vi "Start Sync.vi"(8 "error in (no error)":errorcluster, 11 "gRPC service in":refnum<class "OOBgRPCService.lvclass">) -> (0 "error out":errorcluster, 3 "gRPC service out":refnum<class "OOBgRPCService.lvclass">)   [LabVIEW 2025, in "OOB gRPC Server.lvlib" / "OOBgRPCService.lvclass"]
uses:
  OOBgRPCService.lvclass
  OOBgRPCService.lvclass/OOBgRPCService.ctl
  OOB Data Transfer/OOB Data Transfer.lvlib
  RPC Messages/hwval_GenericResponse.ctl
  OOB gRPC Server.lvlib
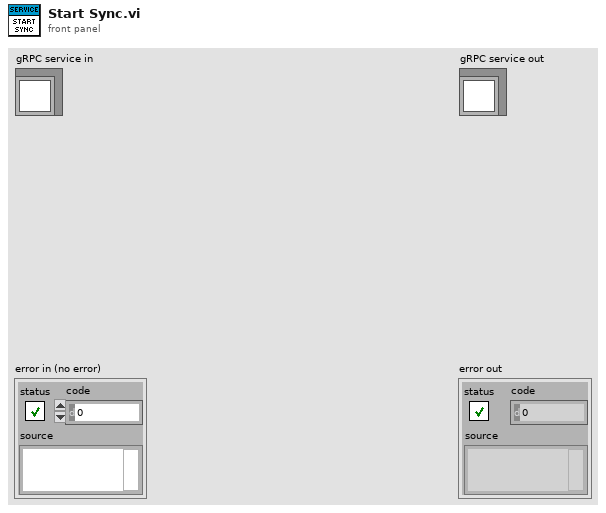
[diagram p1: front panel]
types:
  T1 = typedef "OOB gRPC Server.lvlib/hwval_GenericResponse.ctl" = cluster{"Payload":u8[]}
  T2 = typedef "OOB gRPC Server.lvlib/OOBgRPCService.lvclass/Server Internal UEs.ctl" = cluster{"OOBgRPCService Generic Internal UE":refnum<user-event>, "OOBgRPCService PauseResume Internal UE":refnum<user-event>, "OOBgRPCService Export Internal UE":refnum<user-event>}
  T3 = typedef "OOB gRPC Server.lvlib/OOBgRPCService.lvclass/Server gRPC UEs.ctl" = cluster{"OOBgRPCService Generic gRPC UE":refnum<user-event>, "OOBgRPCService PauseResume gRPC UE":refnum<user-event>, "OOBgRPCService Export gRPC UE":refnum<user-event>}
  T4 = typedef "grpc-lvsupport-release.lvlib/grpcId.ctl" = u64
  T5 = typedef "OOB gRPC Server.lvlib/hwval_GenericRequest.ctl" = cluster{"Command":string, "Payload":u8[]}
  T6 = typedef "OOB gRPC Server.lvlib/hwval_BoolRequest.ctl" = cluster{"BooleanData":bool}
  T7 = typedef "OOB Data Transfer.lvlib/OOB to Logic Data.ctl" = cluster{"PauseResume":bool, "Export":string}
  T8 = typedef "OOB gRPC Server.lvlib/hwval_ExportRequest.ctl" = cluster{"FileType":string}
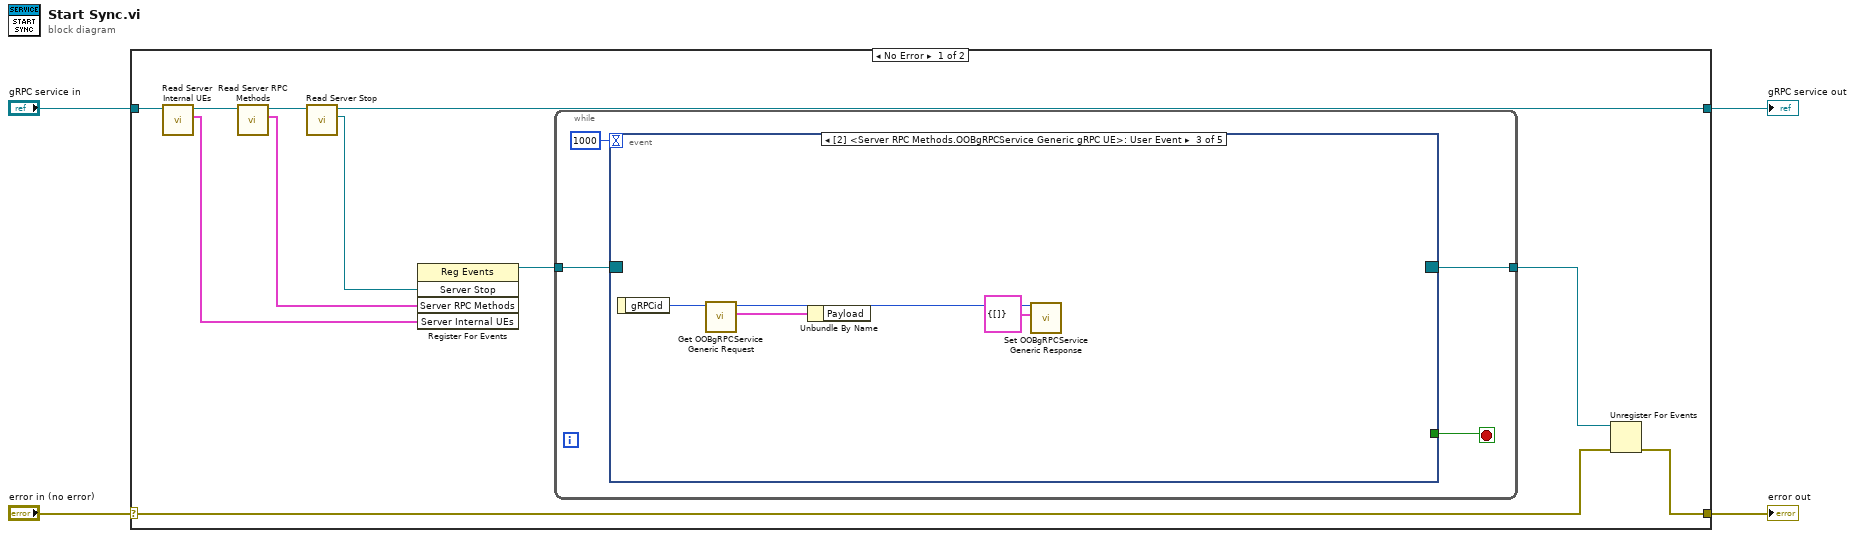
[diagram p0: block diagram]
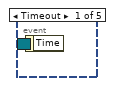
[diagram p2: hidden frame]
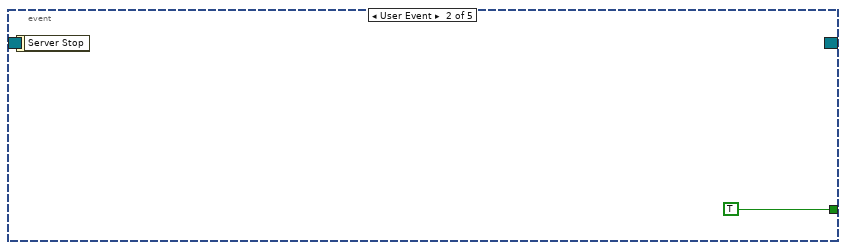
[diagram p3: hidden frame]
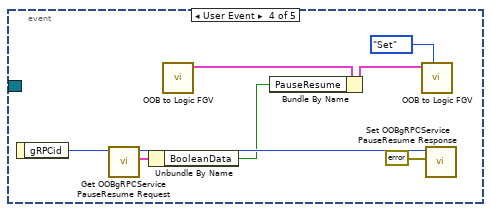
[diagram p4: hidden frame]
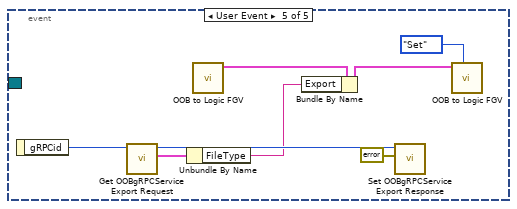
[diagram p5: hidden frame]
diagram:
  n1 = case shown="No Error" "error in (no error)" {
    selector: "error in (no error)" -> [w9 w42]
    tunnel: [w8 w42] -> w3
    tunnel: [w6 w41] -> w1
    tunnel: "gRPC service in" -> [w15 w41]
    frame No Error {
      n2 = call "Read Server Internal UEs.vi"("gRPC service in"=w15) -> ("Server Internal UEs"=w13:T2, "gRPC service out"=w14:refnum<class "OOBgRPCService.lvclass">)  [unwired: 8 in, 1 out]
      n3 = call "Read Server RPC Methods.vi"("gRPC service in"=w14) -> ("Server RPC Methods"=w7:T3, "gRPC service out"=w12:refnum<class "OOBgRPCService.lvclass">)  [unwired: 8 in, 1 out]
      n4 = call-dynamic "Read Server Stop.vi"("gRPC service in"=w12) -> ("Server Stop"=w5:refnum<user-event>, "gRPC service out"=w6:refnum<class "OOBgRPCService.lvclass">)  [unwired: 8 in, 1 out]
      n5 = register-events(w5, w7, w13) -> (reference out=w11:refnum<event-registration>)  [unwired: 2 in, 1 out]
      n6 = while {
        tunnel: w11 -> [w19]
        tunnel: [w17] -> w10
        stop <- w18 stop-if-true
        n7 = event "RPC Methods Event Structure" shown="[2] <Server RPC Methods.OOBgRPCService Generic gRPC UE>: User Event" {
          selector: w19 -> [_ _ _ _ _]
          dyn-events: [_ _ _ _ _] -> w17
          timeout: 1000 -> [_ _ _ _ _]
          tunnel: [_ TRUE _ _ _] -> w18
          event Timeout {
            n8 = event-data() -> ()  [unwired: 1 in, 1 out]
          }
          event User Event {
            n9 = event-data() -> ()  [unwired: 1 in, 1 out]
          }
          event User Event {
            n10 = event-data() -> ("gRPCid"=w24:T4)  [unwired: 1 in]
            n11 = call "Get OOBgRPCService Generic Request.vi"("gRPCid"=w24) -> ("Message Data"=w22:T5, "gRPCid out"=w23:T4)  [unwired: 8 in, 1 out]
            n12 = Unbundle By Name(w22) -> ()  [unwired: 1 out]
            n13 = call "Set OOBgRPCService Generic Response.vi"("Message Data"=T1 {"Payload"=[]}, "gRPCid in"=w23) -> ()  [unwired: 9 in, 1 out]
          }
          event User Event {
            n14 = event-data() -> ("gRPCid"=w25:T4)  [unwired: 1 in]
            n15 = call "Get OOBgRPCService PauseResume Request.vi"("gRPCid"=w25) -> ("Message Data"=w27:T6, "gRPCid out"=w28:T4)  [unwired: 8 in, 1 out]
            n16 = Unbundle By Name(w27) -> ("BooleanData"=w26:bool)
            n17 = call "OOB to Logic FGV.vi"() -> ("OOB to Logic Data out"=w31:T7)  [unwired: 10 in, 1 out]
            n18 = Bundle By Name(cluster=w31, "PauseResume"=w26) -> (w30:T7)
            n19 = call "OOB to Logic FGV.vi"("Op (Get)"=enum16{"Get", "Set"}."Set", "OOB to Logic Data in"=w30) -> ()  [unwired: 8 in, 2 out]
            n20 = call "Set OOBgRPCService PauseResume Response.vi"("Message Data"=errorcluster {"status"=FALSE, "code"=0, "source"=""} ("error in (no error)"), "gRPCid in"=w28) -> ()  [unwired: 9 in, 1 out]
          }
          event User Event {
            n21 = event-data() -> ("gRPCid"=w33:T4)  [unwired: 1 in]
            n22 = call "Get OOBgRPCService Export Request.vi"("gRPCid"=w33) -> ("Message Data"=w35:T8, "gRPCid out"=w40:T4)  [unwired: 8 in, 1 out]
            n23 = Unbundle By Name(w35) -> ("FileType"=w34:string)
            n24 = call "OOB to Logic FGV.vi"() -> ("OOB to Logic Data out"=w37:T7)  [unwired: 10 in, 1 out]
            n25 = Bundle By Name(cluster=w37, "Export"=w34) -> (w36:T7)
            n26 = call "Set OOBgRPCService Export Response.vi"("Message Data"=errorcluster {"status"=FALSE, "code"=0, "source"=""} ("error in (no error)"), "gRPCid in"=w40) -> ()  [unwired: 9 in, 1 out]
            n27 = call "OOB to Logic FGV.vi"("Op (Get)"=enum16{"Get", "Set"}."Set", "OOB to Logic Data in"=w36) -> ()  [unwired: 8 in, 2 out]
          }
        }
      }
      n28 = Unregister For Events(event registration refnum=w10, error in=w9) -> (error out=w8:errorcluster)
    }
    frame Error {
    }
  }
  "error out" <- w3
  "gRPC service out" <- w1
